vi "SPI Engine.Core.Input Buffer 64-bit.vi"(6 "Ready for Output":bool, 9 "Input Valid":bool, 11 "SPI Information In":T1 {"SPI Settings"."SPI Physical Settings"."Direction Change Bit" max=64 step=1; "SPI Settings"."SPI Physical Settings"."Transfer Length (bits)" min=1 max=64 step=1}) -> (1 "Output Valid":bool, 3 "SPI Information Out":T1 {"SPI Settings"."SPI Physical Settings"."Direction Change Bit" max=64 step=1; "SPI Settings"."SPI Physical Settings"."Transfer Length (bits)" min=1 max=64 step=1}, 4 "Ready For Input":bool)   [LabVIEW 2015, in "SPI API.lvlib"]
uses:
  SPI API.lvlib
  Controls/SPI API Transaction Packet 64-bit.ctl
  Controls/SPI API Data 64-bit.ctl
  Controls/SPI Transaction Settings.ctl
  <userlib>/_NI SPI IP/FPGA/Controllers/Public/Transfer Settings.ctl
  <vilib>/rvi/DataTransferAndStorage/Container/Common/niFpgaContainerGetUniqueNameForEmu.vi
  <vilib>/rvi/DataTransferAndStorage/Container/Common/niFpgaContainerSetEmuInfo.vi
  <vilib>/rvi/eio/common/nirviEmuReportErrorAndStop.vi
  <vilib>/rvi/DataTransferAndStorage/Container/Common/niFpgaContainerExecOnDevCompGetState.vi
  <vilib>/rvi/Emulation/niFpgaEmulationIsFPGAContextNoSignature.vi
  <vilib>/rvi/Emulation/niFpgaSctlEmulationGetInTimedLoop.vi
  <vilib>/rvi/errors/niFpgaSetErrorForExecOnDevCompSimple.vi
  <vilib>/rvi/FIFO/Fifo_Resource/nirvififoEmulationSetSize.vi
  <vilib>/rvi/FIFO/Fifo_Resource/nirviFifoEmulationQueueMgr.vi
  <instcachedir>/0/nirviFifoEmulationQueueMgr_E5CAEC123FF24DC58D834DCA3CDAA9B5.lvgen/nirviFifoEmulationQueueMgr_E5CAEC123FF24DC58D834DCA3CDAA9B5_015.vi
  <vilib>/rvi/FIFO/Fifo_Resource/nirvififoEmulationDetermineInputValidOut.vi
  <vilib>/rvi/FIFO/Fifo_Resource/nirvififoEmulationCreateLock.vi
  <vilib>/rvi/Emulation/niFpgaProcessEmulError.vi
  <vilib>/rvi/FIFO/Fifo_Resource/nirvififoEmulationObtainLock.vi
  <vilib>/rvi/FIFO/Fifo_Resource/nirvififoEmulationReleaseLock.vi
  <vilib>/rvi/occurrence/nirviWaitOnOccurrenceBase.vi
  <vilib>/rvi/errors/nirviReportUnexpectedCaseInternalError.vi
  <vilib>/rvi/errors/nirviReportUnexpectedCaseInternalError (U32).vi
  <vilib>/Utility/error.llb/Clear Errors.vi
  <vilib>/rvi/interface/RandomDataEmulation/niFpgaRandomDataHandleErrors.vi
  <vilib>/rvi/LocalResourceManager/LocalResourceManager.xnode
  <vilib>/rvi/DataTransferAndStorage/Container/XNode/niFpgaContainer.xnode
  <vilib>/rvi/FIFO/Fifo_Resource/niFpgaFifoEmulationRefIn.vi
  <userlib>/_NI SPI IP/FPGA/Controllers/NI SPI IP FPGA.lvlib
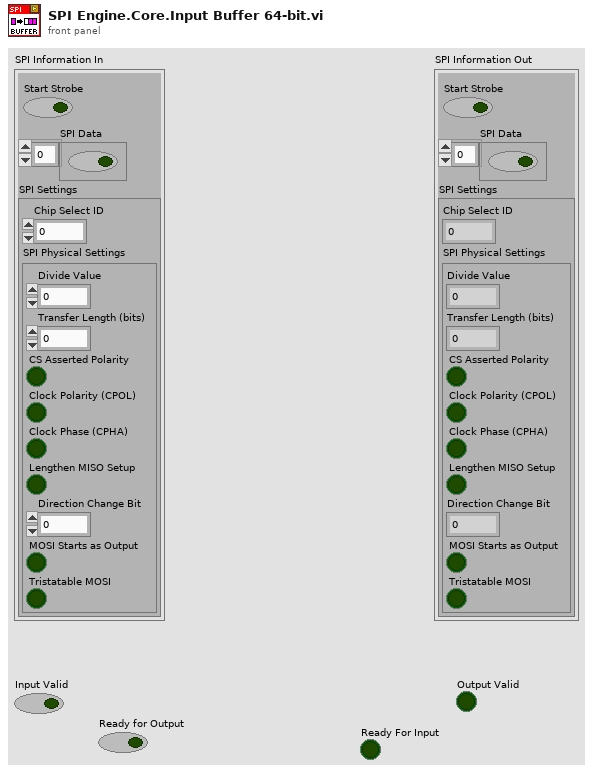
[diagram p1: front panel]
types:
  T1 = typedef "SPI API.lvlib/SPI API Transaction Packet 64-bit.ctl" = cluster{"Start Strobe":bool, "SPI Data":T2, "SPI Settings":T3}
  T2 = typedef "SPI API.lvlib/SPI API Data 64-bit.ctl" = bool[]
  T3 = typedef "SPI API.lvlib/SPI Transaction Settings.ctl" = cluster{"Chip Select ID":u8, "SPI Physical Settings":T4}
  T4 = typedef "NI SPI IP FPGA.lvlib/Transfer Settings.ctl" = cluster{"Divide Value":u8, "Transfer Length (bits)":u8, "CS Asserted Polarity":bool, "Clock Polarity (CPOL)":bool, "Clock Phase (CPHA)":bool, "Lengthen MISO Setup":bool, "Direction Change Bit":u8, "MOSI Starts as Output":bool, "Tristatable MOSI":bool}
  T5 = cluster{"Start Strobe":bool, "Data to Node":bool[], "SPI Settings":cluster{"Chip Select ID":u8, "SPI Physical Settings":cluster{"Divide Value":u8, "Transfer Length (bits)":u8, "CS Asserted Polarity":bool, "Clock Polarity (CPOL)":bool, "Clock Phase (CPHA)":bool, "Lengthen MISO Setup":bool, "Direction Change Bit":u8, "MOSI Starts as Output":bool, "Tristatable MOSI":bool}}}
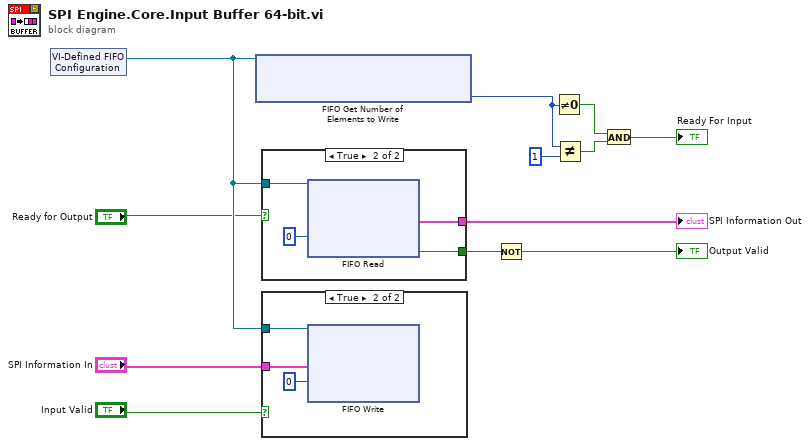
[diagram p0: block diagram]
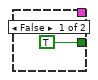
[diagram p2: hidden frame]
diagram:
  n1 = xnode "VI-Defined FIFO Configuration"() -> ("FIFO Out"=w2:refnum<k21>)
  n2 = xnode ("FIFO Get Number of Elements to Write")("FIFO In"=w2) -> ("Number of Elements to Write"=w10:u32)  [unwired: 1 out]
  n3 = case shown="True" "Ready for Output" {
    tunnel: [_ w16] -> w3
    tunnel: [TRUE ("Timed Out?") w15] -> w12
    tunnel: w2 -> [_ w14]
    frame False {
    }
    frame True {
      n4 = xnode ("FIFO Read")("Timeout"=0, "FIFO In"=w14) -> ("Element"=w16:T5, "Timed Out?"=w15:bool)  [unwired: 1 out]
    }
  }
  "SPI Information Out" <- w3
  n5 = case shown="True" "Input Valid" {
    tunnel: "SPI Information In" -> [_ w20]
    tunnel: w2 -> [_ w18]
    frame False {
    }
    frame True {
      n6 = xnode ("FIFO Write")("Element"=w20, "Timeout"=0, "FIFO In"=w18) -> ()  [unwired: 2 out]
    }
  }
  n7 = Not(x=w12) -> (.not. x?=→"Output Valid":bool)
  n8 = Not Equal To 0?(x=w10) -> (x != 0?=w8:bool)
  n9 = Not Equal?(x=w10, y=u32 1) -> (x != y?=w9:bool)
  n10 = And(x=w8, y=w9) -> (x .and. y?=→"Ready For Input":bool)
